vi "registerAllEvents.vi"(8 "error in (no error)":errorcluster, 11 "Monochromator in":refnum<class "Monochromator.lvclass">) -> (0 "error out":errorcluster, 2 "AllEventsRegRefnum":refnum<event-registration>, 3 "Monochromator out":refnum<class "Monochromator.lvclass">)   [LabVIEW 2020, in "Monochromator.lvclass"]
uses:
  Monochromator.lvclass
  Typedefs/slit.ctl
  Typedefs/SlitType.ctl
  Typedefs/slitWidth.ctl
  Typedefs/GratingType.ctl
  Typedefs/wavelength.ctl
  Monochromator.lvclass/Monochromator.ctl
  MonoPubSubData/MonoPubSubData.lvclass
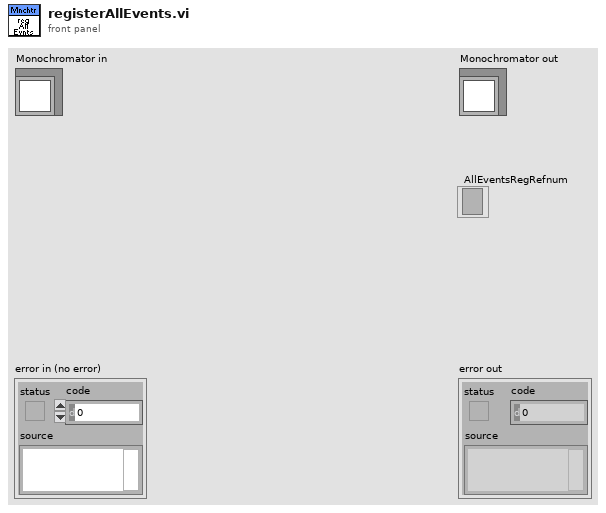
[diagram p1: front panel]
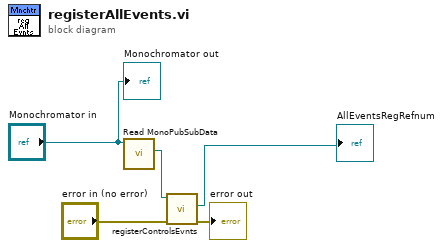
[diagram p0: block diagram]
diagram:
  n1 = call "Read MonoPubSubData.vi"("Monochromator in"="Monochromator in") -> ("MonoPubSubData.lvclass"=w4:refnum<class "MonoPubSubData.lvclass">)  [unwired: 8 in, 2 out]
  n2 = call "registerControlsEvnts.vi"("error in (no error)"="error in (no error)", "MonoPubSubData in"=w4) -> ("error out"=→"error out":errorcluster, "AllEventsRegRefnum"=→"AllEventsRegRefnum":refnum<event-registration>)  [unwired: 7 in, 1 out]
  "Monochromator out" <- "Monochromator in"
